vi "RTMain.vi"() -> ()   [LabVIEW 2022 SP3]
uses:
  <vilib>/rvi/interface/RandomDataEmulation/nirviRandomDataOpen.vi
  <vilib>/rvi/interface/common/niFpgaCacheSessionInfoDynamic.vi
  <vilib>/Utility/error.llb/Error Cluster From Error Code.vi
  <vilib>/rvi/errors/niLvFpgaAdjustHostInterfaceError.vi
  <vilib>/FPGAPlugInAG/Dynamic/niLvFpga_Close_Dynamic.vi
  <vilib>/rvi/interface/nirviOpenFPGA/nirviOpenFPGA.xnode
  FPGAMain.vi
  <vilib>/rvi/interface/nirviMethod/nirviMethod.xnode
  <vilib>/rvi/interface/nirviCloseFPGA/nirviCloseFPGA.xnode
  <vilib>/FPGAPlugInAG/Dynamic/niLvFpga_WriteFifo_Dynamic.vi
  <vilib>/rvi/errors/niLvFpgaMergeErrorWithErrorCode.vi
  <vilib>/FPGAPlugInAG/Dynamic/niLvFpga_ReadFifo_Dynamic.vi
panel:
  out "bytes written":i32
  out "data sent":i16[](array[numeric])
  out "buffer":i16[](array[numeric])
  out "buffer size":i32
  out "FIFO read error":errorcluster
  out "FPGA ref error":errorcluster
  out "TCP client send error":errorcluster
  out "Control Signals":bool[](array[boolean])
  out "TCP client receive error":errorcluster
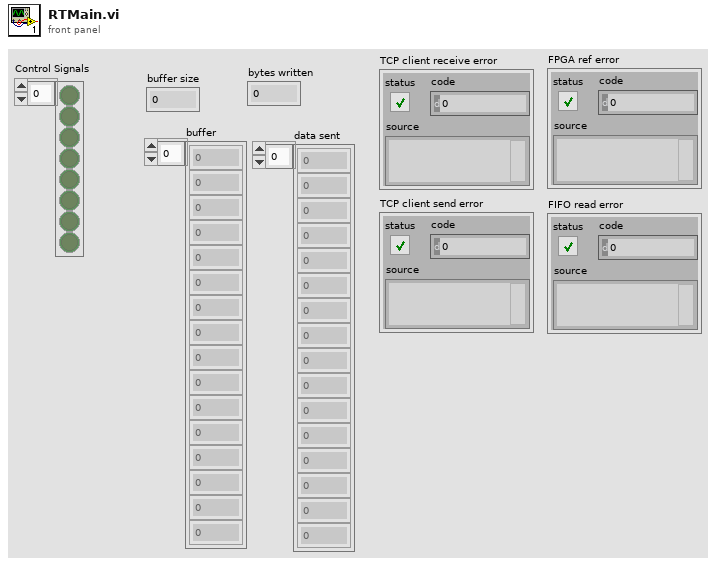
[diagram p1: front panel]
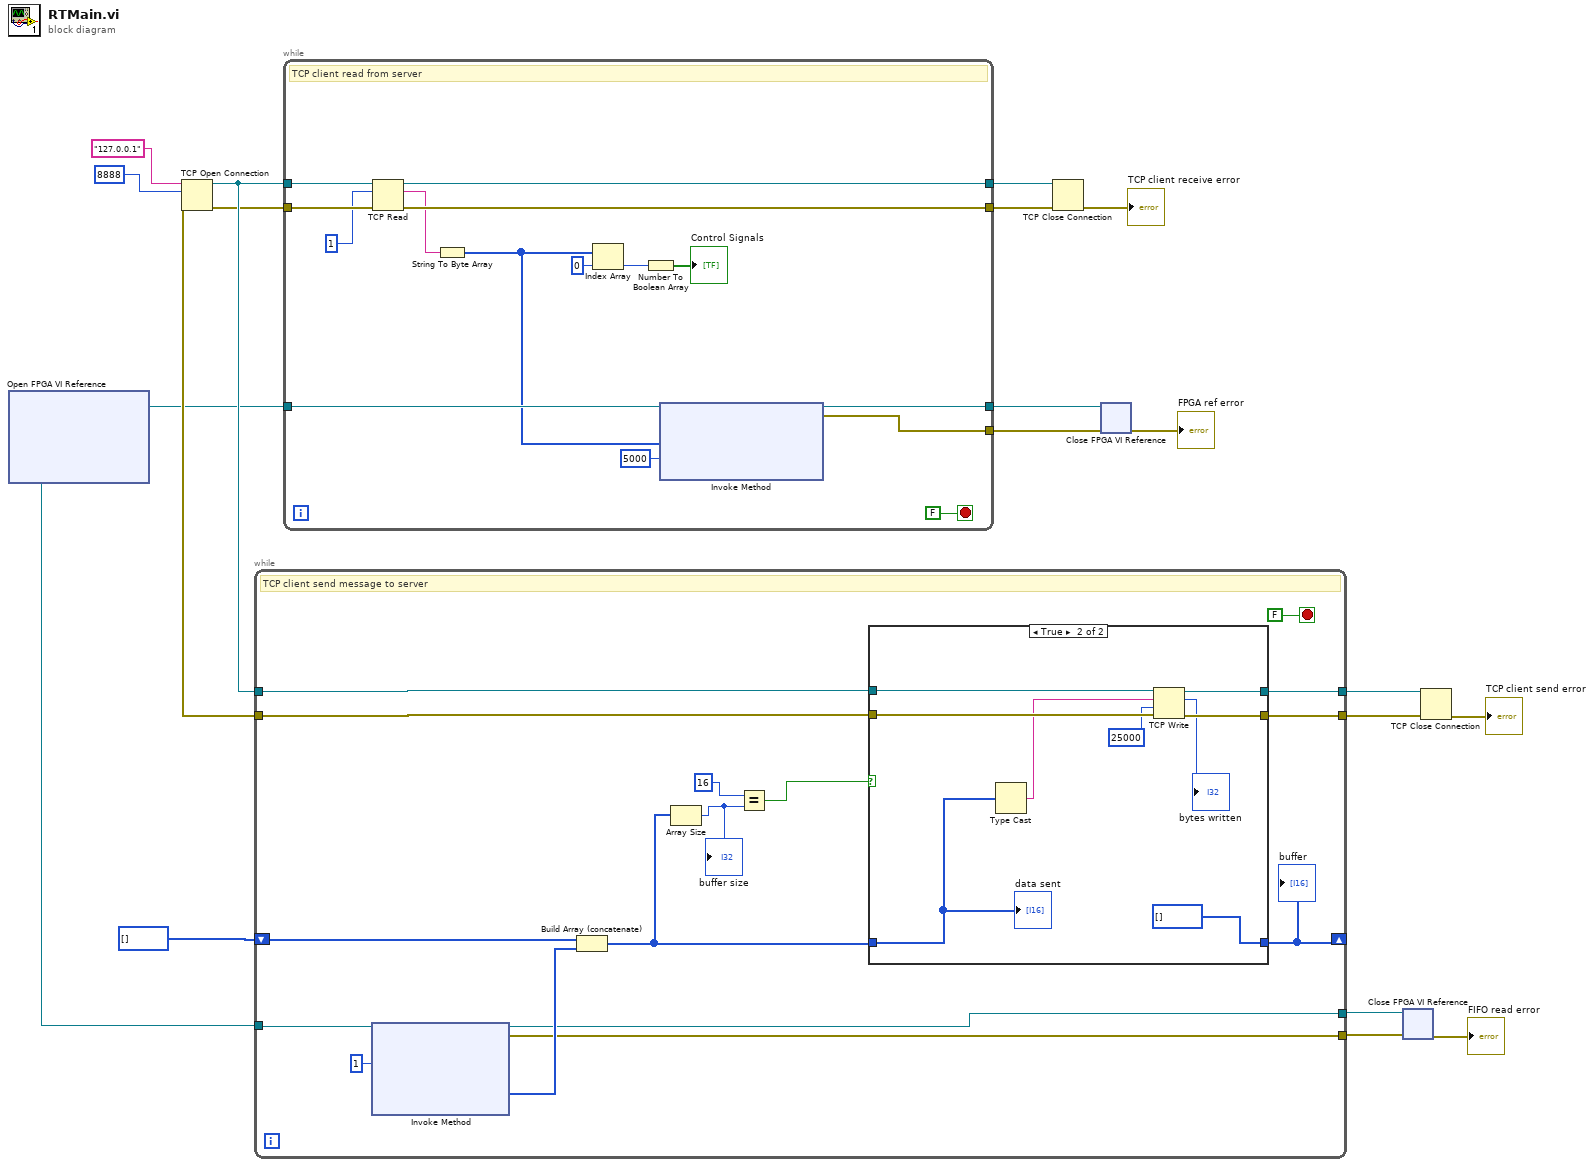
[diagram p0: block diagram]
diagram:
  n1 = xnode "Open FPGA VI Reference"() -> ("FPGA VI Reference Out"=w5:refnum<k20>)  [unwired: 2 in, 1 out]
  n2 = TCP Open Connection(address="127.0.0.1", remote port or service name=u16 8888) -> (connection ID=w13:refnum<k5>, error out=w12:errorcluster)  [unwired: 3 in]
  n3 = while {
    tunnel: w13 -> [w33]
    tunnel: w12 -> [w32]
    tunnel: [w31] -> w10
    tunnel: [w30] -> w9
    tunnel: w5 -> [w25]
    shift-right: [w20] -> _
    shift-left: i16[] [] -> [w24]
    tunnel: [w22] -> w3
    tunnel: [w21] -> w2
    stop <- FALSE stop-if-true
    # "TCP client send message to server"
    n4 = xnode "Invoke Method"("FPGA VI Reference In"=w25, "Number of Elements"=u32 1) -> ("FPGA VI Reference Out"=w22:refnum<k20>, "error out"=w21:errorcluster, "Data"=w28:i16[])  [unwired: 2 in, 1 out]
    n5 = Build Array (concatenate)(w24, w28) -> (w19:i16[])
    n6 = Array Size(array=w19) -> (size(s)=w29:i32)
    "buffer size" <- w29
    n7 = Equal?(x=16, y=w29) -> (x = y?=w23:bool)
    n8 = case shown="True" w23 {
      tunnel: w33 -> [w37 w46]
      tunnel: w32 -> [w36 w45]
      tunnel: [w37 w44] -> w31
      tunnel: [w36 w43] -> w30
      tunnel: [w35 i16[] []] -> w20
      tunnel: w19 -> [w35 w39]
      frame False {
      }
      frame True {
        n9 = Type Cast(x=w39) -> (*(type *) &x=w38:string)  [unwired: 1 in]
        n10 = TCP Write(connection ID=w46, data in=w38, error in (no error)=w45, 9:25000 ("timeout ms (25000)")) -> (connection ID out=w44:refnum<k5>, bytes written=→"bytes written":i32, error out=w43:errorcluster)
        "data sent" <- w39
      }
    }
    "buffer" <- w20
  }
  n11 = while {
    tunnel: w13 -> [w61]
    tunnel: w12 -> [w60]
    tunnel: [w57] -> w16
    tunnel: [w56] -> w15
    tunnel: w5 -> [w52]
    tunnel: [w49] -> w8
    tunnel: [w48] -> w7
    stop <- FALSE stop-if-true
    # "TCP client read from server"
    n12 = TCP Read(connection ID=w61, bytes to read=1, error in (no error)=w60) -> (connection ID out=w57:refnum<k5>, data out=w55:string, error out=w56:errorcluster)  [unwired: 2 in]
    n13 = String To Byte Array(string=w55) -> (unsigned byte array=w50:u8[])
    n14 = Index Array(array=w50, index=0) -> (element=w51:u8)
    n15 = Number To Boolean Array(number=w51) -> (Boolean array=→"Control Signals":bool[])
    n16 = xnode "Invoke Method"("FPGA VI Reference In"=w52, "Data"=w50, "Timeout (ms)"=5000) -> ("FPGA VI Reference Out"=w49:refnum<k20>, "error out"=w48:errorcluster)  [unwired: 1 in, 1 out]
  }
  n17 = TCP Close Connection(connection ID=w16, error in (no error)=w15) -> (error out=→"TCP client receive error":errorcluster)  [unwired: 1 in, 1 out]
  n18 = xnode "Close FPGA VI Reference"("FPGA VI Reference In"=w8, "error in"=w7) -> ("error out"=→"FPGA ref error":errorcluster)
  n19 = xnode "Close FPGA VI Reference"("FPGA VI Reference In"=w3, "error in"=w2) -> ("error out"=→"FIFO read error":errorcluster)
  n20 = TCP Close Connection(connection ID=w10, error in (no error)=w9) -> (error out=→"TCP client send error":errorcluster)  [unwired: 1 in, 1 out]
